vi "Functional data-Generate dummy data.vi"(7 "Trial number (unity-based)":i32=1 min=1, 9 "total no. of points in each cycle":i32=10, 11 "no. of  cycles":i32=1) -> (3 "Single trial data (inc. POIs and miniscans, multiple cycles)":u32[](graph))   [LabVIEW 2013]
panel:
  out "Total data points per channel":i32
  out "Channel B":u32[](graph)
  out "Channel A":u32[](graph)
  out "Total data points across both channels":i32
  # "Includes each an every individual miniscan point plus all POI points."
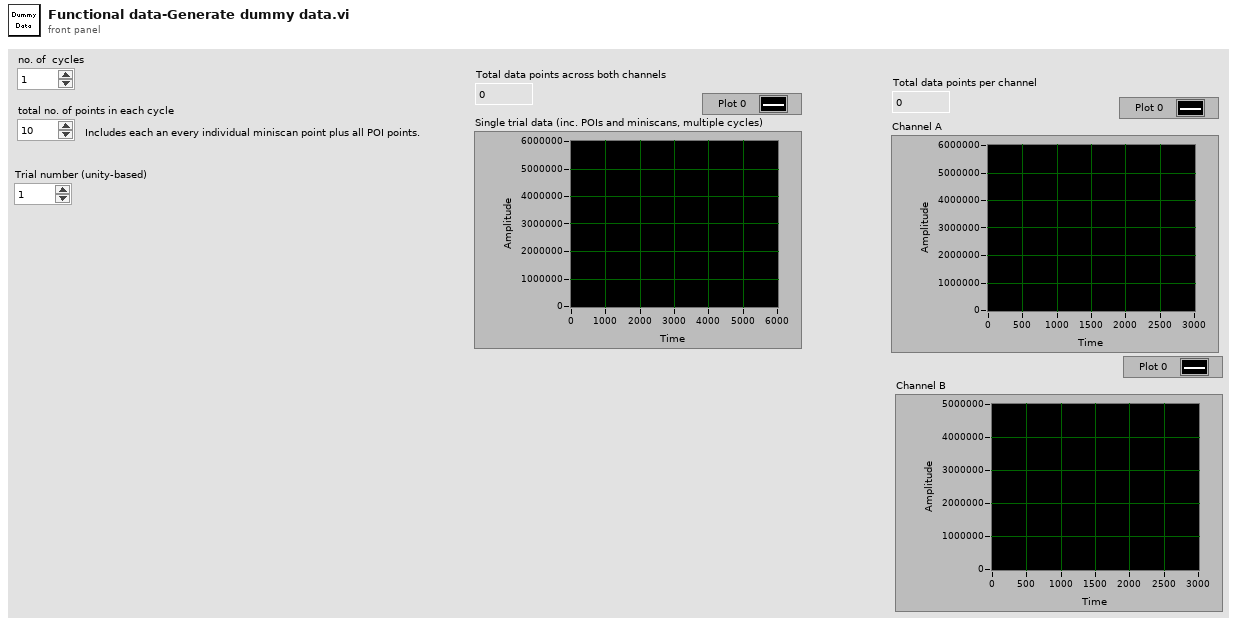
[diagram p1: front panel]
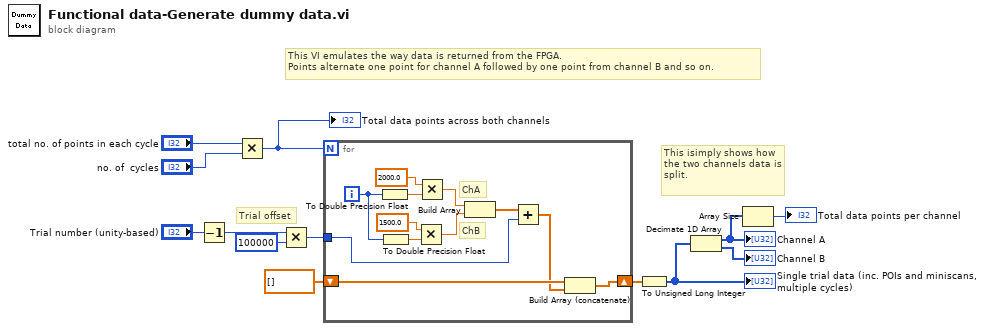
[diagram p0: block diagram]
diagram:
  # "Trial offset"
  # "This isimply shows how the two channels data is split."
  # "This VI emulates the way data is returned from the FPGA.\nPoints alternate one point for channel A followed by one point from channel B and so on."
  n1 = Decrement(x="Trial number (unity-based)") -> (x-1=w1:i32)
  n2 = Multiply(x="total no. of points in each cycle", y="no. of  cycles") -> (x*y=w11:i32)
  "Total data points across both channels" <- w11
  n3 = Multiply(x=w1, y=100000) -> (x*y=w2:i32)
  n4 = for {
    N: w11 -> [_]
    shift-right: [w17] -> w9
    shift-left: dbl[] [] -> [w18]
    tunnel: w2 -> [w14]
    i -> [w21]
    # "ChB"
    # "ChA"
    n5 = To Double Precision Float(number=w21) -> (double precision float=w24:dbl)
    n6 = To Double Precision Float(number=w21) -> (double precision float=w23:dbl)
    n7 = Multiply(x=1500.0, y=w23) -> (x*y=w19:dbl)
    n8 = Multiply(x=2000.0, y=w24) -> (x*y=w20:dbl)
    n9 = Build Array(w20, w19) -> (w16:dbl[])
    n10 = Add(x=w16, y=w14) -> (x+y=w15:dbl[])
    n11 = Build Array (concatenate)(w18, w15) -> (w17:dbl[])
  }
  n12 = To Unsigned Long Integer(number=w9) -> (unsigned 32bit integer=w8:u32[])
  "Single trial data (inc. POIs and miniscans, multiple cycles)" <- w8
  n13 = Decimate 1D Array(w8) -> (w6:u32[], →"Channel B":u32[])
  "Channel A" <- w6
  n14 = Array Size(array=w6) -> (size(s)=→"Total data points per channel":i32)
